vi "Read HW Status.vi"(8 "error in (no error)":errorcluster, 11 "General Hardware in":refnum<class "General Hardware.lvclass">) -> (0 "error out":errorcluster, 2 "shutdown?":bool, 3 "General Hardware out":refnum<class "General Hardware.lvclass">)   [LabVIEW 2020, in "General Hardware.lvclass"]
uses:
  General Hardware.lvclass
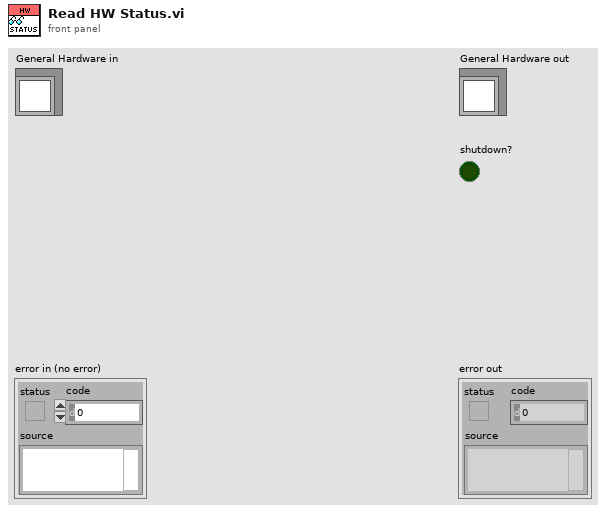
[diagram p1: front panel]
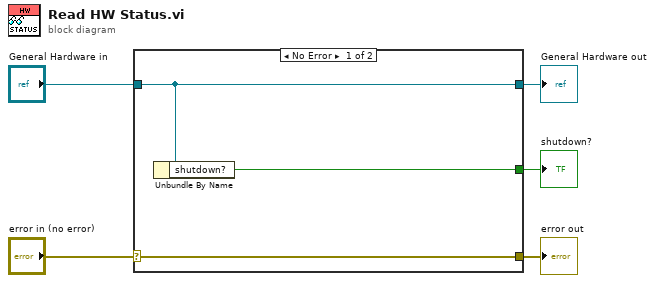
[diagram p0: block diagram]
diagram:
  n1 = case shown="No Error" "error in (no error)" {
    selector: "error in (no error)" -> [w8 w9]
    tunnel: [w8 w9] -> w4
    tunnel: [w7 w10] -> w2
    tunnel: "General Hardware in" -> [w7 w10]
    tunnel: [w6 _] -> w1
    frame No Error {
      n2 = Unbundle By Name(w7) -> ("shutdown?"=w6:bool)
    }
    frame Error {
    }
  }
  "error out" <- w4
  "General Hardware out" <- w2
  "shutdown?" <- w1
